vi "USB_CAN_MakeCANID.vi"(2 "ID":u32 format="%04x", 4 "ExtFrame":bool) -> (5 "IDS":u8[](array[numeric]) format="%02x")   [LabVIEW 2011]
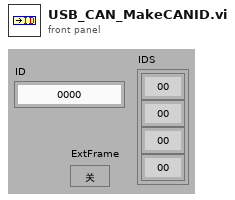
[diagram p1: front panel]
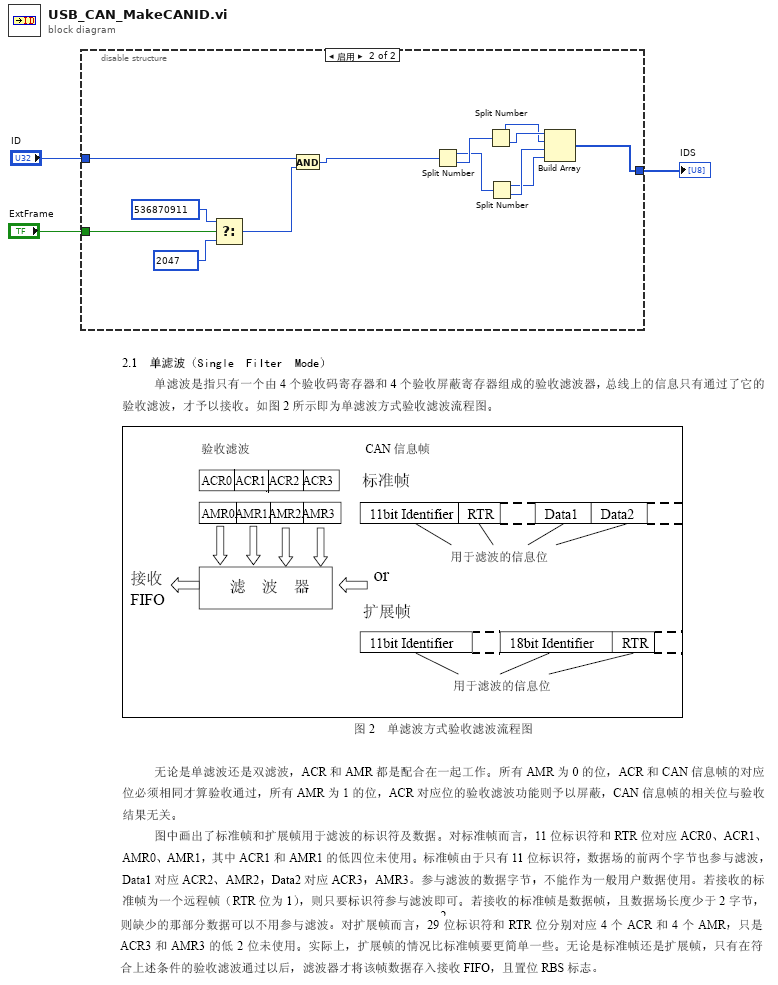
[diagram p0: block diagram]
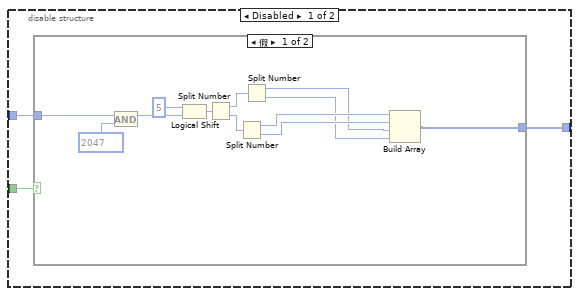
[diagram p2: hidden frame]
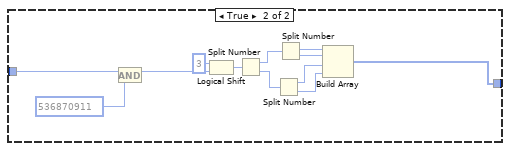
[diagram p3: hidden frame]
diagram:
  n1 = disable-structure shown="启用" {
    disable-tunnel: "ID" -> [w6 w39]
    disable-tunnel: [w5 w31] -> w2
    disable-tunnel: "ExtFrame" -> [w4 w41]
    frame Disabled {
      n2 = case shown="假" w4 {
        tunnel: w6 -> [w18 w30]
        tunnel: [w10 w21] -> w5
        frame False {
          n3 = And(x=w18, y=u32 2047) -> (x .and. y?=w16:u32)
          n4 = Logical Shift(y=i8 5, x=w16) -> (x << y=w14:u32)
          n5 = Split Number(x=w14) -> (hi(x)=w9:u16, lo(x)=w13:u16)
          n6 = Split Number(x=w13) -> (hi(x)=w12:u8, lo(x)=w11:u8)
          n7 = Split Number(x=w9) -> (hi(x)=w7:u8, lo(x)=w8:u8)
          n8 = Build Array(w12, w11, w7, w8) -> (w10:u8[])
        }
        frame True {
          n9 = And(x=w30, y=u32 536870911) -> (x .and. y?=w20:u32)
          n10 = Logical Shift(y=i8 3, x=w20) -> (x << y=w28:u32)
          n11 = Split Number(x=w28) -> (hi(x)=w27:u16, lo(x)=w26:u16)
          n12 = Split Number(x=w26) -> (hi(x)=w23:u8, lo(x)=w22:u8)
          n13 = Split Number(x=w27) -> (hi(x)=w25:u8, lo(x)=w24:u8)
          n14 = Build Array(w25, w24, w23, w22) -> (w21:u8[])
        }
      }
    }
    frame Enabled {
      n15 = Select(t=u32 536870911 ("y"), s=w41, f=u32 2047 ("y")) -> (s? t:f=w40:u32)
      n16 = And(x=w39, y=w40) -> (x .and. y?=w32:u32)
      n17 = Split Number(x=w32) -> (hi(x)=w37:u16, lo(x)=w38:u16)
      n18 = Split Number(x=w38) -> (hi(x)=w35:u8, lo(x)=w36:u8)
      n19 = Split Number(x=w37) -> (hi(x)=w33:u8, lo(x)=w34:u8)
      n20 = Build Array(w36, w35, w34, w33) -> (w31:u8[])
    }
  }
  "IDS" <- w2
